vi "Threshold Color2.vi"(2 "Luma Range":cluster{"Lower value":i32, "Upper value":i32}={"Lower value"=0, "Upper value"=255}, 3 "Sat Range":cluster{"Lower value":i32, "Upper value":i32}={"Lower value"=0, "Upper value"=255}, 4 "error in (no error)":errorcluster, 5 "Hue Range":cluster{"Lower value":i32, "Upper value":i32}={"Lower value"=0, "Upper value"=255}, 6 "Image Dst":T1, 7 "Image Src":T1) -> (0 "error out":errorcluster, 1 "Image Dst Out":T1)   [LabVIEW 2009, in "ImageProcessing.lvlib"]
doc: "Thresholds a grayscaled image and does som clean up"
uses:
  ImageProcessing.lvlib
  <vilib>/vision/Image Controls.llb/IMAQ Image.ctl
  <vilib>/vision/NI_Vision_Development_Module.lvlib
panel:
  out "Thresholded Image":T1(plugin-control) caption="HSL Threshold"
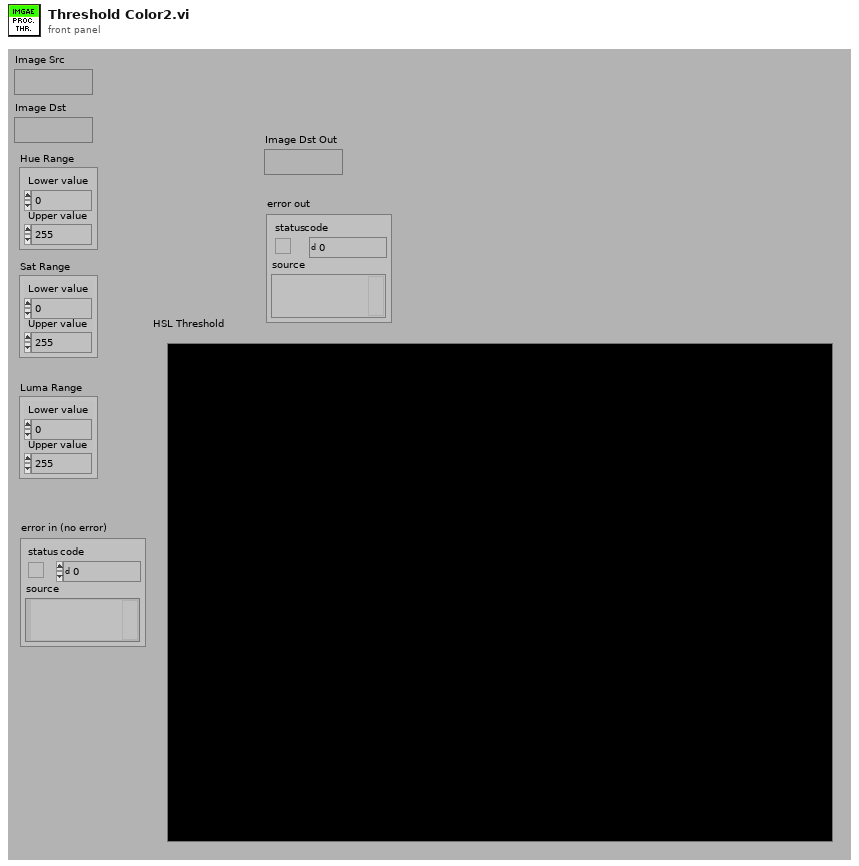
[diagram p1: front panel]
types:
  T1 = typedef "IMAQ Image.ctl" = refnum<image>
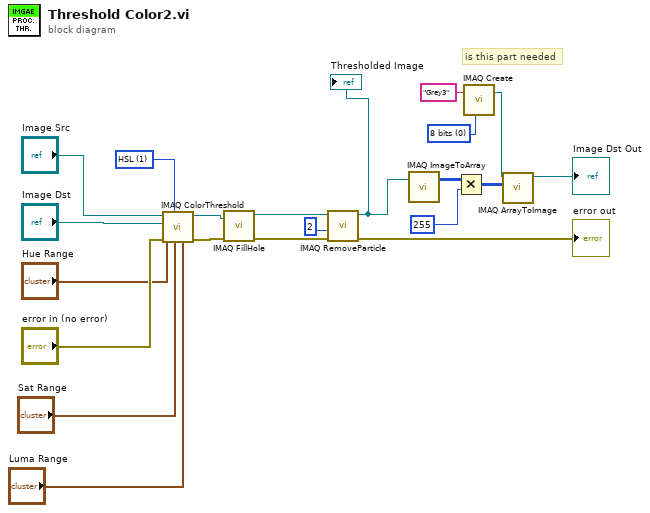
[diagram p0: block diagram]
diagram:
  w8 = u16 1 items=["RGB", "HSL", "HSV", "HSI"] ("Color Mode")
  w14 = u32 0 items=["8 bits", "16 bits", "Float", "Complex", "RGB", "HSL"] ("Image Type")
  # "is this part needed"
  n1 = call "IMAQ ColorThreshold"("Blue or Luma or Val or Inten Range"="Luma Range", "Green or Sat Range"="Sat Range", "Color Mode"=w8, "error in (no error)"="error in (no error)", "Red or Hue Range"="Hue Range", "Image Dst"="Image Dst", "Image Src"="Image Src") -> ("error out"=w6:errorcluster, "Image Dst Out"=w2:T1)  [unwired: 3 in]
  n2 = call "IMAQ FillHole"("error in (no error)"=w6, "Image Src"=w2) -> ("error out"=w20:errorcluster, "Image Dst Out"=w19:T1)  [unwired: 2 in, 2 out]
  n3 = call "IMAQ RemoveParticle"("error in (no error)"=w20, "Number of Erosion"=2, "Image Src"=w19) -> ("error out"=→"error out":errorcluster, "Image Dst Out"=w1:T1)  [unwired: 4 in, 3 out]
  "Thresholded Image" <- w1
  n4 = call "IMAQ ImageToArray"("Image"=w1) -> ("Image Pixels (U8)"=w18:u8[][])  [unwired: 3 in, 4 out]
  n5 = Multiply(x=w18, y=255) -> (x*y=w16:i32[][])
  n6 = call "IMAQ Create"("Image Name"="Grey3", "Image Type"=w14) -> ("New Image"=w13:T1)  [unwired: 2 in, 2 out]
  n7 = call "IMAQ ArrayToImage"("Image Pixels (U8)"=w16, "Image"=w13) -> ("Image Out"=→"Image Dst Out":T1)  [unwired: 8 in, 1 out]
